vi "Initialize File.vi"(6 "wait for reply (T)":bool=TRUE, 8 "error in (no error)":errorcluster) -> (0 "error out":errorcluster, 1 "timed out?":bool, 2 "Reply Payload":T1)   [LabVIEW 2020, in "Logger.lvlib"]
doc: "Request the Logger to initialize the file and report when the Logger has initialized the file.\n_____\nCreated using Delacor QMH Event Scripter 4.1.0.75.\n_____\nBased on DQMH Project Template 6.0.0.91."
uses:
  Logger.lvlib
  Initialize File (Reply Payload)--cluster.ctl
  Initialize File Argument--cluster.ctl
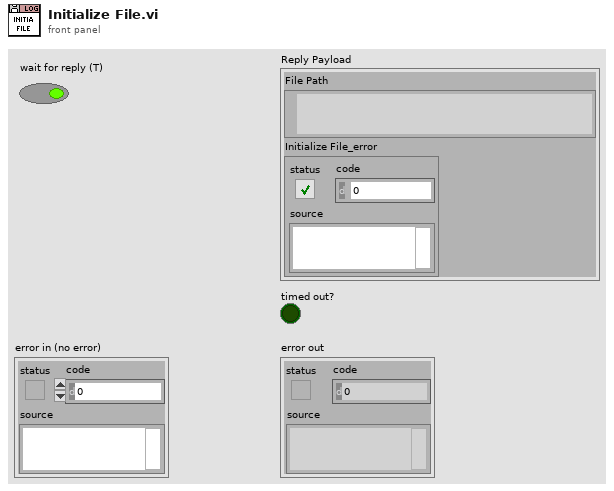
[diagram p1: front panel]
types:
  T1 = typedef "Logger.lvlib/Initialize File (Reply Payload)--cluster.ctl" = cluster{"File Path":path, "Initialize File_error":errorcluster}
  T2 = typedef "Logger.lvlib/Initialize File Argument--cluster.ctl" = cluster{"Wait Notifier":refnum<notifier>, "wait for reply":bool}
  T3 = typedef "Logger.lvlib/Request Events--cluster.ctl" = cluster{"Stop Module":refnum<user-event>, "Show Panel":refnum<user-event>, "Hide Panel":refnum<user-event>, "Get Module Execution Status":refnum<user-event>, "Show Diagram":refnum<user-event>, "Stop Logging":refnum<user-event>, "Log Data":refnum<user-event>, "Initialize File":refnum<user-event>}
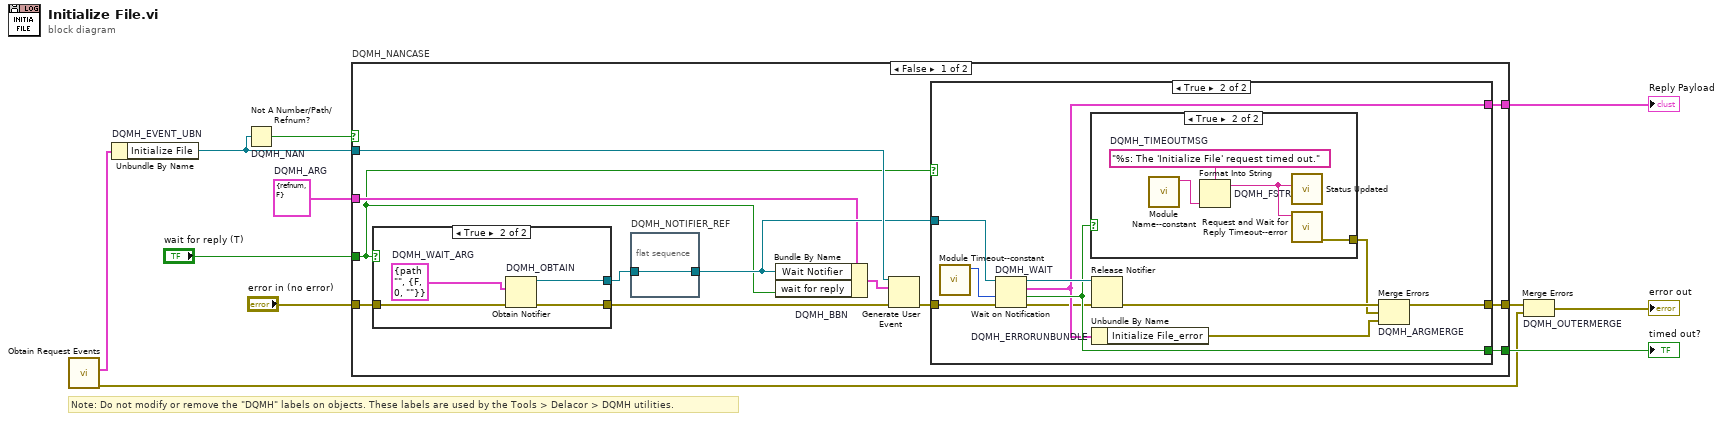
[diagram p0: block diagram]
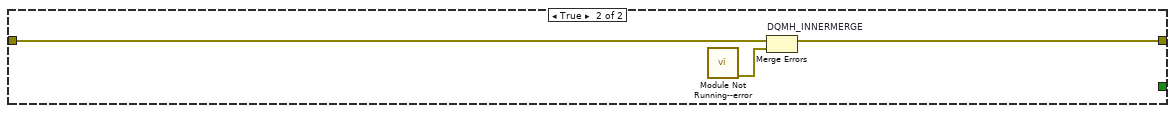
[diagram p5: hidden frame]
diagram:
  w5 = T2 {"Wait Notifier"=refnum, "wait for reply"=FALSE}  # DQMH_ARG
  # "Note: Do not modify or remove the \"DQMH\" labels on objects. These labels are used by the Tools > Delacor > DQMH utilities."
  n1 = call "Obtain Request Events.vi"() -> ("error out"=w3:errorcluster, "Logger Request Events"=w2:T3)  [unwired: 10 in]
  n2 = Unbundle By Name "DQMH_EVENT_UBN"(w2) -> ("Initialize File"=w9:refnum<user-event>)
  n3 = Not A Number/Path/Refnum? "DQMH_NAN"(number/path/refnum=w9) -> (NaN/Path/Refnum?=w8:bool)
  n4 = case "DQMH_NANCASE" shown="False" w8 {
    tunnel: "error in (no error)" -> [w23 w48]
    tunnel: w9 -> [w21 _]
    tunnel: [w18 w47] -> w6
    tunnel: [w19 _] -> w7
    tunnel: w5 -> [w14 _]
    tunnel: "wait for reply (T)" -> [w13 _]
    tunnel: [w12 _] -> w1
    frame False {
      n5 = case shown="True" w13 {
        tunnel: w23 -> [w41 w45]
        tunnel: [w41 w44] -> w20
        tunnel: [_ w42] -> w16
        frame False {
        }
        frame True {
          w43 = T1 {"File Path"=path "", "Initialize File_error"={"status"=FALSE, "code"=0, "source"=""}}  # DQMH_WAIT_ARG
          n6 = Obtain Notifier "DQMH_OBTAIN"(notification data type=w43, error in (no error)=w45) -> (notifier out=w42:refnum<notifier>, error out=w44:errorcluster)  [unwired: 2 in, 1 out]
        }
      }
      n7 = flat-sequence "DQMH_NOTIFIER_REF" {
        tunnel: w16 -> [w24]
        tunnel: [w24] -> w15
        frame #0 {
        }
      }
      n8 = Bundle By Name "DQMH_BBN"(cluster=w14, "Wait Notifier"=w15, "wait for reply"=w13) -> (w17:T2)
      n9 = Generate User Event(user event=w21, event data cluster=w17, error in=w20) -> (error out=w22:errorcluster)  [unwired: 1 in, 1 out]
      n10 = case shown="True" w13 {
        tunnel: w22 -> [w25 w36]
        tunnel: w15 -> [_ w35]
        tunnel: [_ w33] -> w19
        tunnel: [w25 w32] -> w18
        tunnel: [_ w30] -> w12
        frame False {
        }
        frame True {
          n11 = call "Module Timeout--constant.vi"() -> ("Module Timeout"=w31:i32)  [unwired: 11 in]
          n12 = Wait on Notification "DQMH_WAIT"(notifier=w35, timeout in ms (-1)=w31, error in (no error)=w36) -> (notifier out=w34:refnum<notifier>, notification=w30:T1, timed out?=w33:bool, error out=w29:errorcluster)  [unwired: 1 in]
          n13 = case shown="True" w33 {
            tunnel: [_ w38] -> w26
            frame False {
            }
            frame True {
              w40 = "%s: The 'Initialize File' request timed out."  # DQMH_TIMEOUTMSG
              n14 = call "Module Name--constant.vi"() -> ("Module Name"=w39:string)  [unwired: 11 in]
              n15 = Format Into String "DQMH_FSTR"(format string=w40, w39) -> (resulting string=w37:string)  [unwired: 2 in, 1 out]
              n16 = call "Status Updated.vi"("Status"=w37) -> ()  [unwired: 10 in, 1 out]
              n17 = call "Request and Wait for Reply Timeout--error.vi"("Error Message"=w37) -> ("error out"=w38:errorcluster)  [unwired: 10 in]
            }
          }
          n18 = Release Notifier(notifier=w34, error in (no error)=w29) -> (error out=w28:errorcluster)  [unwired: 1 in, 2 out]
          n19 = Unbundle By Name "DQMH_ERRORUNBUNDLE"(w30) -> ("Initialize File_error"=w27:errorcluster)
          n20 = Merge Errors "DQMH_ARGMERGE"(w28, w26, w27) -> (w32:errorcluster)
        }
      }
    }
    frame True {
      n21 = call "Module Not Running--error.vi"() -> ("error out"=w46:errorcluster)  [unwired: 11 in]
      n22 = Merge Errors "DQMH_INNERMERGE"(w48, w46) -> (w47:errorcluster)
    }
  }
  "timed out?" <- w7
  "Reply Payload" <- w1
  n23 = Merge Errors "DQMH_OUTERMERGE"(w6, w3) -> (→"error out":errorcluster)
